vi "get_RegArrAndTimeout.vi"(4 "error in (no error)":errorcluster, 7 "HGF_SVMonitor":refnum<class "HGF_SVMonitor.lvclass">) -> (0 "error out":errorcluster, 1 "Registration Array":T1(array[cluster]), 2 "timeout in ms(10)":i32, 3 "HGF_SVMonitor":refnum<class "HGF_SVMonitor.lvclass">)   [LabVIEW 2012, in "HGF_SV.lvlib" / "HGF_SVMonitor.lvclass"]
doc: "Get registration array, timeout and comparison method selection from monitor object"
uses:
  HGF_SVMonitor.lvclass
  HGF_BaseClasses/HGF_NetworkVisitor/HGF_NetworkVisitor.lvclass
  HGF_BaseClasses/HGF_TriggeredEvent/HGF_TriggeredEvent.lvclass
  HGF_SVMonitor.lvclass/HGF_SVMonitor.ctl
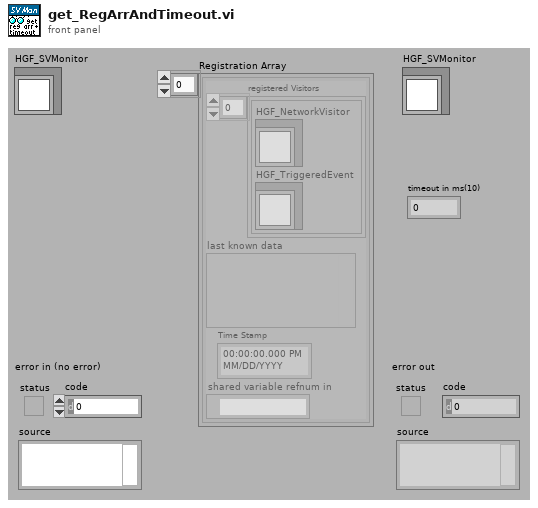
[diagram p1: front panel]
types:
  T1 = cluster{"registered Visitors":cluster{"HGF_NetworkVisitor":refnum<class "HGF_NetworkVisitor.lvclass">, "HGF_TriggeredEvent":refnum<class "HGF_TriggeredEvent.lvclass">}[], "last known data":variant, "Time Stamp":timestamp, "shared variable refnum in":refnum<k21>}[]
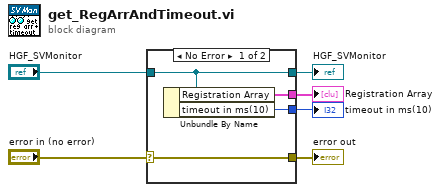
[diagram p0: block diagram]
diagram:
  n1 = case shown="No Error" "error in (no error)" {
    selector: "error in (no error)" -> [w10 w11]
    tunnel: [w10 w11] -> w5
    tunnel: [w9 w12] -> w3
    tunnel: "HGF_SVMonitor" -> [w9 w12]
    tunnel: [w8 _] -> w2
    tunnel: [w7 _] -> w1
    frame No Error {
      n2 = Unbundle By Name(w9) -> ("Registration Array"=w7:T1, "timeout in ms(10)"=w8:i32)
    }
    frame Error {
    }
  }
  "error out" <- w5
  "HGF_SVMonitor" <- w3
  "timeout in ms(10)" <- w2
  "Registration Array" <- w1
